vi "GetTestDistWithDotRange.vi"(8 "错误输入（无错误）":errorcluster) -> (0 "错误输出":errorcluster, 3 "返回值":sgl)   [LabVIEW 2014]
uses:
  X86Dll/ZXUTConfigMgr.dll
panel:
  in  "采样点位置":u16
  in  "当前通道序号":u8
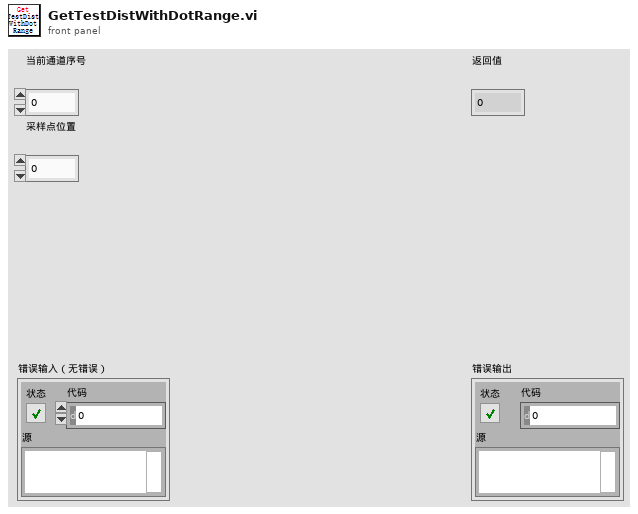
[diagram p1: front panel]
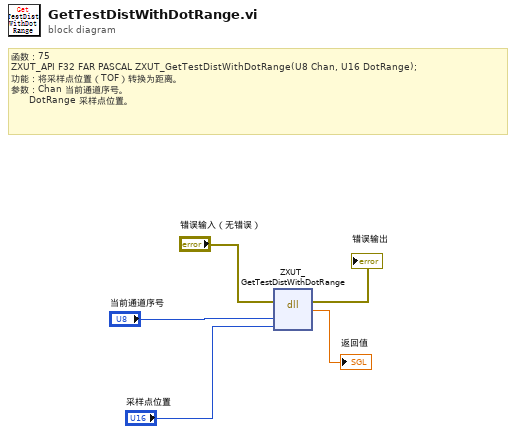
[diagram p0: block diagram]
diagram:
  # "函数：75\nZXUT_API F32\tFAR PASCAL ZXUT_GetTestDistWithDotRange(U8 Chan, U16 DotRange);\n功能：将采样点位置（TOF）转换为距离。\n参数：Chan 当前通道序号。\n      DotRange 采样点位置。"
  n1 = dll-call lib="D:/Software/Utrasonic on-line monitoring/X86Dll/ZXUTConfigMgr.dll" fn="ZXUT_GetTestDistWithDotRange"(error in="错误输入（无错误）", "Chan"="当前通道序号", "DotRange"="采样点位置") -> (error out=→"错误输出":errorcluster, "返回值"=→"返回值":sgl)  [unwired: 4 in, 1 out]
